vi "get Polynoms of all Komponents.vi"(11 "Komponente":T1) -> (3 "Polynom Array":string[](array[string]))   [LabVIEW 2020, in "Linearisierung v2.lvlib"]
uses:
  Linearisierung v2.lvlib
  Visualisierungs Elemente/Auswahlfeld.ctl
  Aktionen Polynom Daten speichern.ctl
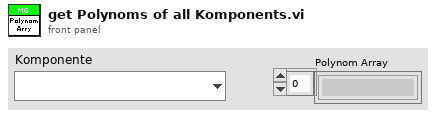
[diagram p1: front panel]
types:
  T1 = typedef "Auswahlfeld.ctl" = u16
  T2 = typedef "Linearisierung v2.lvlib/Aktionen Polynom Daten speichern.ctl" = enum16{"lesen", "laden", "speichern", "schreiben", "schreiben alle", "Liste erstellen", "aktivieren", "deaktivieren", "aktiv abfragen"}
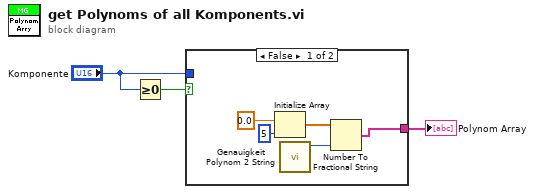
[diagram p0: block diagram]
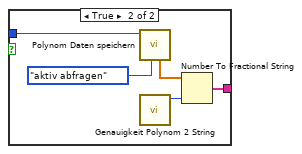
[diagram p2: hidden frame]
diagram:
  n1 = Greater Or Equal To 0?(x="Komponente") -> (x >= 0?=w2:bool)
  n2 = case shown="False" w2 {
    tunnel: "Komponente" -> [_ w10]
    tunnel: [w5 w9] -> w3
    frame False {
      n3 = Initialize Array(0.0 ("Numerisch"), 5 ("Dimensionsgröße")) -> (w6:dbl[])
      n4 = call "Genauigkeit Polynom 2 String.vi"() -> ("Genauigkeit Polynom 2 String"=w4:i16)  [unwired: 9 in, 2 out]
      n5 = Number To Fractional String(number=w6, precision (6)=w4) -> (F-format string=w5:string[])  [unwired: 2 in]
    }
    frame True {
      n6 = call "Polynom Daten speichern.vi"("Aktionen"=Aktionen_Polynom_Daten_speichern."aktiv abfragen", "Komponente"=w10) -> ("Einzelnes Polynom out"=w13:dbl[])  [unwired: 4 in, 5 out]
      n7 = call "Genauigkeit Polynom 2 String.vi"() -> ("Genauigkeit Polynom 2 String"=w12:i16)  [unwired: 9 in, 2 out]
      n8 = Number To Fractional String(number=w13, precision (6)=w12) -> (F-format string=w9:string[])  [unwired: 2 in]
    }
  }
  "Polynom Array" <- w3
